vi "A33ConfigureWFM.vi"(4 "Frequency/BW/BitRate (1000.0 Hz)":dbl=1000.0 format="%#_12g", 5 "Phase (0 deg)":dbl format="%#_12g", 6 "DC Offset (0.0 Volts)":dbl step=0.01 format="%#_12g", 7 "Waveform (0: Sine)":u16(ring) items=["Sine", "Square", "Pulse", "Ramp", "Noise", "DC", "PRBS", "Triangle"], 8 "error in (no error)":errorcluster, 9 "Amplitude (1.0 Vpp)":dbl=1.0 format="%#_12g", 10 "Channel (1: Channel1)":u16(ring)=1 items=["Channel1"=1, "Channel2"=2], 11 "VISA resource name":refnum<visa-resource-name>) -> (0 "error out":errorcluster, 3 "VISA resource name out":refnum<visa-resource-name>)   [LabVIEW 2022 SP3]
doc: "Selects the waveform shape, frequency, amplitude, offset, and phase for a standard waveform."
panel:
  # "-For ARB waveforms use separte vi\n-Pulse period,width,edges - separate vi\n-Noise/PRBS - seprate vi"
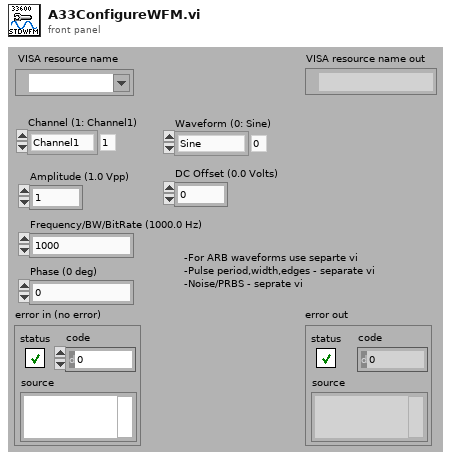
[diagram p1: front panel]
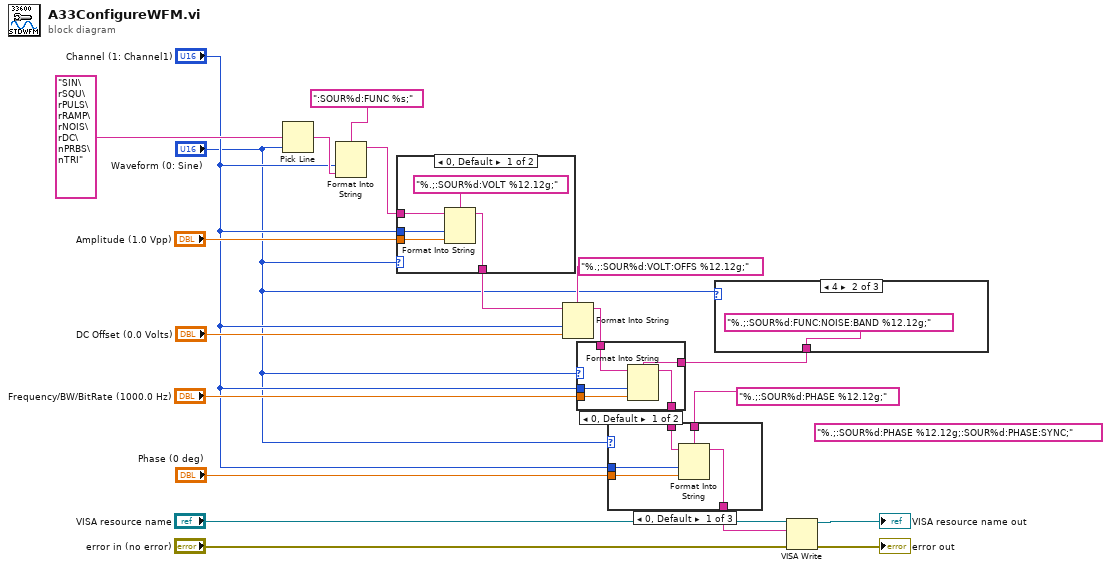
[diagram p0: block diagram]
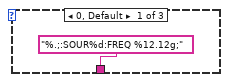
[diagram p6: hidden frame]
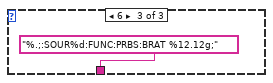
[diagram p7: hidden frame]
diagram:
  (unwired) "%.;:SOUR%d:PHASE %12.12g;:SOUR%d:PHASE:SYNC;"
  n1 = Pick Line(multi-line string="SIN\rSQU\rPULS\rRAMP\rNOIS\rDC\nPRBS\nTRI", line index="Waveform (0: Sine)") -> (output string=w19:string)  [unwired: 1 in]
  n2 = Format Into String(format string=":SOUR%d:FUNC %s;", "Channel (1: Channel1)", w19) -> (resulting string=w8:string)  [unwired: 2 in, 1 out]
  n3 = case shown="0, Default" "Waveform (0: Sine)" {
    tunnel: "Amplitude (1.0 Vpp)" -> [w25 _]
    tunnel: [w24 w27] -> w16
    tunnel: w8 -> [w23 w27]
    tunnel: "Channel (1: Channel1)" -> [w22 _]
    frame 0, Default {
      n4 = Format Into String(format string="%.;:SOUR%d:VOLT %12.12g;", initial string=w23, w22, w25) -> (resulting string=w24:string)  [unwired: 1 in, 1 out]
    }
    frame 5 {
    }
  }
  n5 = Format Into String(format string="%.;:SOUR%d:VOLT:OFFS %12.12g;", initial string=w16, "Channel (1: Channel1)", "DC Offset (0.0 Volts)") -> (resulting string=w14:string)  [unwired: 1 in, 1 out]
  n6 = case shown="4" "Waveform (0: Sine)" {
    tunnel: ["%.;:SOUR%d:FREQ %12.12g;" "%.;:SOUR%d:FUNC:NOISE:BAND %12.12g;" "%.;:SOUR%d:FUNC:PRBS:BRAT %12.12g;"] -> w7
    frame 0, Default {
    }
    frame 4 {
    }
    frame 6 {
    }
  }
  n7 = case shown="0, Default" "Waveform (0: Sine)" {
    tunnel: w14 -> [w35 w36]
    tunnel: "Frequency/BW/BitRate (1000.0 Hz)" -> [w34 _]
    tunnel: w7 -> [w33 _]
    tunnel: [w32 w36] -> w6
    tunnel: "Channel (1: Channel1)" -> [w31 _]
    frame 0, Default {
      n8 = Format Into String(format string=w33, initial string=w35, w31, w34) -> (resulting string=w32:string)  [unwired: 1 in, 1 out]
    }
    frame 5 {
    }
  }
  n9 = case shown="0, Default" "Waveform (0: Sine)" {
    tunnel: w6 -> [w41 w42 w43]
    tunnel: [w40 w42 w43] -> w5
    tunnel: "Phase (0 deg)" -> [w39 _ _]
    tunnel: "%.;:SOUR%d:PHASE %12.12g;" -> [w38 _ _]
    tunnel: "Channel (1: Channel1)" -> [w37 _ _]
    frame 0, Default {
      n10 = Format Into String(format string=w38, initial string=w41, w37, w39) -> (resulting string=w40:string)  [unwired: 1 in, 1 out]
    }
    frame 4 {
    }
    frame 5 {
    }
  }
  n11 = VISA Write(VISA resource name="VISA resource name", write buffer=w5, error in (no error)="error in (no error)") -> (VISA resource name out=→"VISA resource name out":refnum<visa-resource-name>, error out=→"error out":errorcluster)  [unwired: 1 out]
